vi "Read Analogue.vi"(8 "error in (no error)":errorcluster, 11 "Hioki BT4560B":refnum<class "Hioki BT4560B.lvclass">) -> (0 "error out":errorcluster, 2 "Waveforms":waveform(dbl)[](array[waveform]), 3 "Hioki BT4560B out":refnum<class "Hioki BT4560B.lvclass">)   [LabVIEW 2025, in "ACIR.lvlib" / "Hioki BT4560B.lvclass"]
uses:
  Hioki BT4560B.lvclass
  Hioki BT4560B.lvclass/Hioki BT4560B.ctl
  <instrlib>/HIOKI BT4560/HIOKI BT4560.lvlib
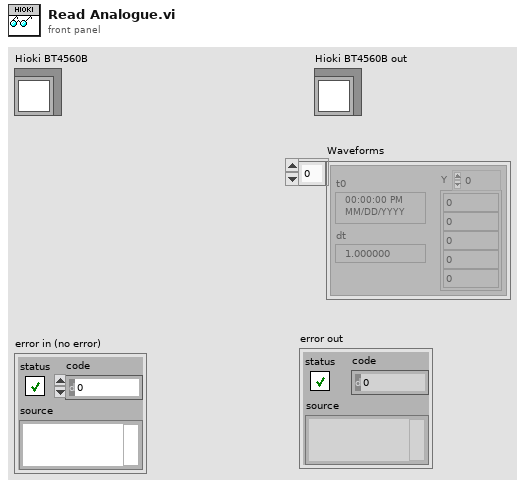
[diagram p1: front panel]
types:
  T1 = typedef "Abstract Engine.lvlibp/Abstract Instrument.lvclass/Channel.ctl" = cluster{"Alias":string, "DataType":enum16{"Anaolg Input", "Waveform"}, "Unit":enum16{"---", "V", "A", "Ohm", "Hz", "uF", "degC", "deg"}, "Upper limit":dbl, "Lower limit":dbl, "Measurement":variant}
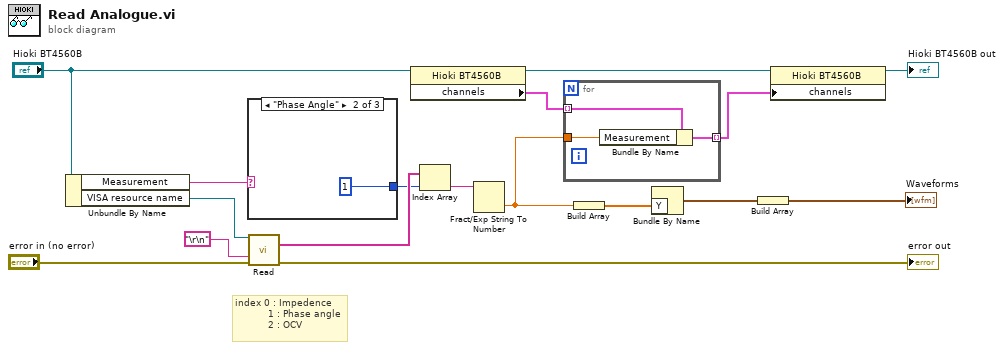
[diagram p0: block diagram]
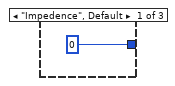
[diagram p2: hidden frame]
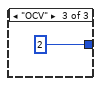
[diagram p3: hidden frame]
diagram:
  # "index 0 : Impedence\n           1 : Phase angle\n           2 : OCV"
  n1 = Unbundle By Name("Hioki BT4560B") -> ("Measurement"=w12:string, "VISA resource name"=w14:refnum<visa-resource-name>)
  n2 = case shown="\"Phase Angle\"" w12 {
    tunnel: [0 1 2] -> w10
    frame "Impedence", Default {
    }
    frame "Phase Angle" {
    }
    frame "OCV" {
    }
  }
  n3 = call <instrlib>:"Read.vi"("VISA session"=w14, "Terminator"="\r\n", "error in (no error)"="error in (no error)") -> ("Output Str"=w11:string[], "error out"=→"error out":errorcluster)  [unwired: 9 in, 2 out]
  n4 = property class="Hioki BT4560B"(reference="Hioki BT4560B") -> (reference out=w8:refnum<class "Hioki BT4560B.lvclass">, "channels"=w6:T1[])  [unwired: 1 in, 1 out]
  n5 = Index Array(array=w11, index=w10) -> (element=w9:string)
  n6 = Fract/Exp String To Number(string=w9) -> (number=w5:dbl)  [unwired: 3 in, 1 out]
  n7 = for {
    tunnel: w6 -> [w21] mode=indexing
    tunnel: [w23] -> w4 mode=indexing
    tunnel: w5 -> [w22]
    n8 = Bundle By Name(cluster=w21, "Measurement"=w22) -> (w23:T1)
  }
  n9 = Build Array(w5) -> (w3:dbl[])
  n10 = Bundle By Name("Y"=w3) -> (w2:waveform(dbl))  [unwired: 1 in]
  n11 = Build Array(w2) -> (→"Waveforms":waveform(dbl)[])
  n12 = property class="Hioki BT4560B"(reference=w8, "channels"=w4) -> (reference out=→"Hioki BT4560B out":refnum<class "Hioki BT4560B.lvclass">)  [unwired: 1 in, 1 out]
